vi "inst.InitialiseFGV.vi"(8 "error in (no error)":errorcluster) -> (0 "error out":errorcluster)   [LabVIEW 2018, in "MB Relay.lvlib"]
uses:
  MB Relay.lvlib
  type defs/FGV enum.ctl
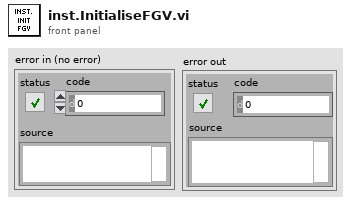
[diagram p1: front panel]
types:
  T1 = typedef "MB Relay.lvlib/FGV enum.ctl" = enum16{"Write", "Init FGV", "Read", "All OFF", "All ON"}
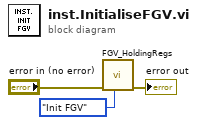
[diagram p0: block diagram]
diagram:
  n1 = call "FGV_HoldingRegs.vi"("FGV_enum"=FGV_enum."Init FGV", "error in (no error)"="error in (no error)") -> ("error out"=→"error out":errorcluster)  [unwired: 7 in, 2 out]
